vi "Measurement Logic.vi"() -> ()   [LabVIEW 2020, in "Game Of Life.lvlib"]
uses:
  Game Of Life.lvlib
  Measurement Results.ctl
  <vilib>/numeric/Random Number (Range) U64.vi
  <vilib>/gRPC/Generated APIs/ni/protobuf/types/RPC Messages/ni_protobuf_types_DoubleXYData.ctl
  <vilib>/MeasurementLink/MeasurementLink Measurement Server/Measure Call Context/Measure Call Context.lvclass
  Measurement Configuration.ctl
panel:
  out "Measurement Context out":refnum<class "Measure Call Context.lvclass">
  in  "Measurement Context":refnum<class "Measure Call Context.lvclass">
  out "Measurement Results":T1
  in  "Measurement Configuration":T3
  out "error out":errorcluster
  in  "error in":errorcluster
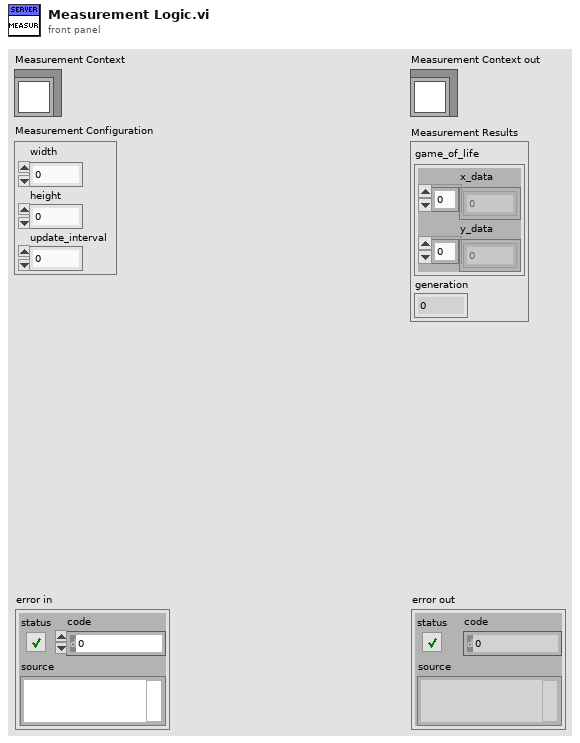
[diagram p1: front panel]
types:
  T1 = typedef "Game Of Life.lvlib/Measurement Results.ctl" = cluster{"game_of_life":T2, "generation":u32}
  T2 = typedef "ni.protobuf.types.lvlib/ni_protobuf_types_DoubleXYData.ctl" = cluster{"x_data":dbl[], "y_data":dbl[]}
  T3 = typedef "Game Of Life.lvlib/Measurement Configuration.ctl" = cluster{"width":u32, "height":u32, "update_interval":u32}
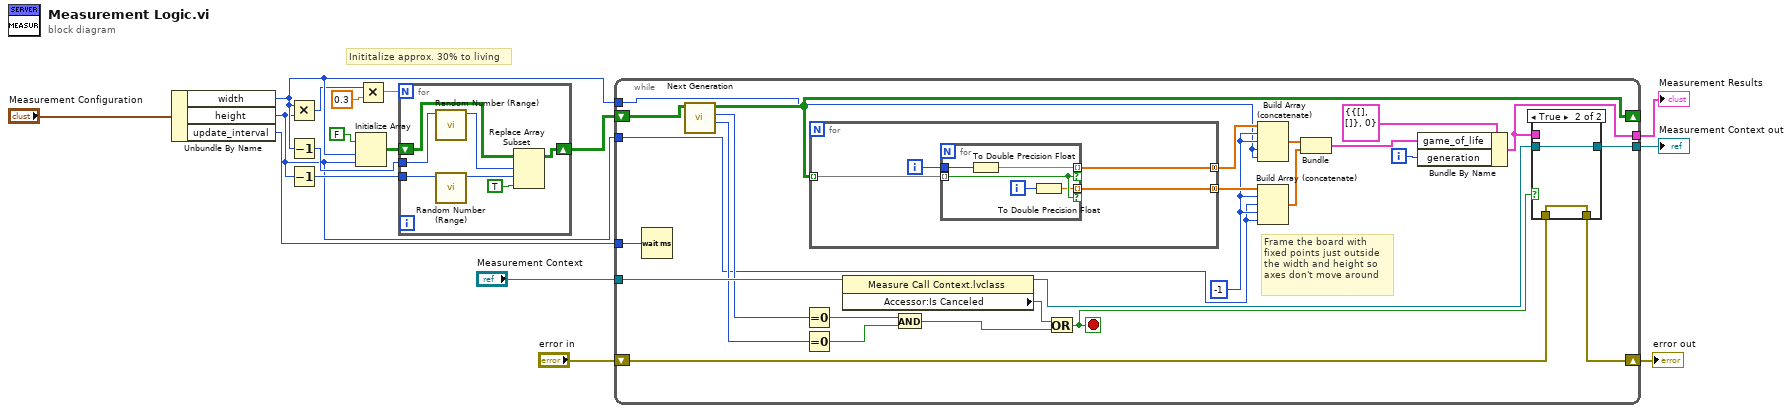
[diagram p0: block diagram]
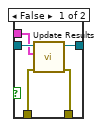
[diagram p2: hidden frame]
diagram:
  # "Inititalize approx. 30% to living"
  n1 = Unbundle By Name("Measurement Configuration") -> ("width"=w8:u32, "height"=w7:u32, "update_interval"=w13:u32)
  n2 = Multiply(x=w8, y=w7) -> (x*y=w6:u32)
  n3 = Decrement(x=w8) -> (x-1=w11:u32)
  n4 = Decrement(x=w7) -> (x-1=w10:u32)
  n5 = Initialize Array(FALSE, w8, w7) -> (w9:bool[][])
  n6 = Multiply(x=w6, y=0.3) -> (x*y=w4:dbl)
  n7 = for {
    N: w4 -> [_]
    tunnel: w11 -> [w24]
    tunnel: w10 -> [w23]
    shift-right: [w18] -> w3
    shift-left: w9 -> [w22]
    n8 = call-poly <vilib>:"Random Number (Range).vi"("upper bound (100)"=w24) -> ("number"=w21:u64)  [unwired: 10 in]
    n9 = call-poly <vilib>:"Random Number (Range).vi"("upper bound (100)"=w23) -> ("number"=w20:u64)  [unwired: 10 in]
    n10 = Replace Array Subset(array=w22, new element=TRUE ("new element/subarray"), index (row)=w21, index (col)=w20) -> (w18:bool[][])
  }
  n11 = while {
    shift-right: [w43] -> _
    shift-left: w3 -> [w50]
    tunnel: "Measurement Context" -> [w48]
    tunnel: [w46] -> w15
    tunnel: [w44] -> w14
    tunnel: w13 -> [w41]
    tunnel: w8 -> [w30]
    tunnel: w7 -> [w29]
    shift-right: [w27] -> w1
    shift-left: "error in" -> [w28]
    i -> [w42]
    stop <- w40 stop-if-true
    w31 = -1
    # "Frame the board with\nfixed points just outside\nthe width and height so\naxes don't move around"
    n12 = Wait (ms)(milliseconds to wait=w41) -> ()  [unwired: 1 out]
    n13 = call "Next Generation.vi"("cells in"=w50) -> ("deaths"=w38:i32, "births"=w39:i32, "cells out"=w43:bool[][])  [unwired: 8 in]
    n14 = Equal To 0?(x=w39) -> (x = 0?=w37:bool)
    n15 = Equal To 0?(x=w38) -> (x = 0?=w36:bool)
    n16 = for {
      tunnel: w43 -> [w61] mode=indexing
      tunnel: [w59] -> w35 mode=concatenating
      tunnel: [w58] -> w33 mode=concatenating
      i -> [w60]
      n17 = for {
        tunnel: w61 -> [w66] mode=indexing
        tunnel: [w64] -> w59 mode=indexing if=w66
        tunnel: w60 -> [w65]
        tunnel: [w62] -> w58 mode=indexing if=w66
        i -> [w63]
        n18 = To Double Precision Float(number=w65) -> (double precision float=w64:dbl)
        n19 = To Double Precision Float(number=w63) -> (double precision float=w62:dbl)
      }
    }
    n20 = property class="Measure Call Context.lvclass"(reference=w48) -> (reference out=w47:refnum<class "Measure Call Context.lvclass">, "Accessor:Is Canceled"=w26:bool)  [unwired: 1 in, 1 out]
    n21 = And(x=w37, y=w36) -> (x .and. y?=w25:bool)
    n22 = Or(x=w26, y=w25) -> (x .or. y?=w40:bool)
    n23 = Build Array (concatenate)(w35, w31, w31, w30, w30) -> (w34:dbl[])
    n24 = Build Array (concatenate)(w33, w31, w29, w31, w29) -> (w32:dbl[])
    n25 = Bundle(w34, w32) -> (w45:cluster{dbl[], dbl[]})  [unwired: 1 in]
    n26 = Bundle By Name(cluster=T1 {"game_of_life"={"x_data"=[], "y_data"=[]}, "generation"=0} ("Measurement Results"), "game_of_life"=w45, "generation"=w42) -> (w44:T1)
    n27 = case shown="True" w40 {
      tunnel: w47 -> [w55 w57]
      tunnel: [w54 w57] -> w46
      tunnel: w44 -> [w53 _]
      tunnel: w28 -> [w52 w56]
      tunnel: [w51 w56] -> w27
      frame False {
        n28 = call <vilib>:"Update Results.vi"("error in (no error)"=w52, "Measurement Results"=w53, "MeasurementContext in"=w55) -> ("error out"=w51:errorcluster, "MeasurementContext out"=w54:refnum<class "Measure Call Context.lvclass">)  [unwired: 7 in]
      }
      frame True {
      }
    }
  }
  "error out" <- w1
  "Measurement Results" <- w14
  "Measurement Context out" <- w15
